vi "TestExplorer.vi"() -> ()   [LabVIEW 2019, in "TestExplorer.lvlib"]
uses:
  TestExplorer.lvlib
  TestResult/TestResult.lvclass
  TestRunner/TestRunner.lvclass
  ResultTreeListener/ResultTreeListener.lvclass
  C:/Users/de200256/Code/neuperger/lvunit/TestListener/TestListener.lvclass
  ResultTree/ResultTree.lvclass
panel:
  out "#Total":i32
  out "#Failed":i32
  out "#Passed":i32
  in  "Result Tree":string(tree)
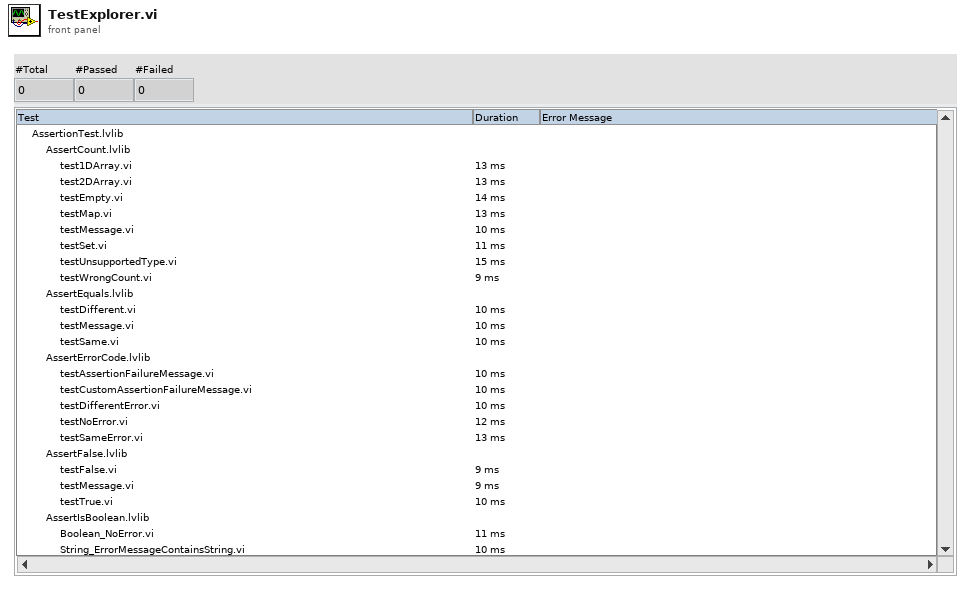
[diagram p1: front panel]
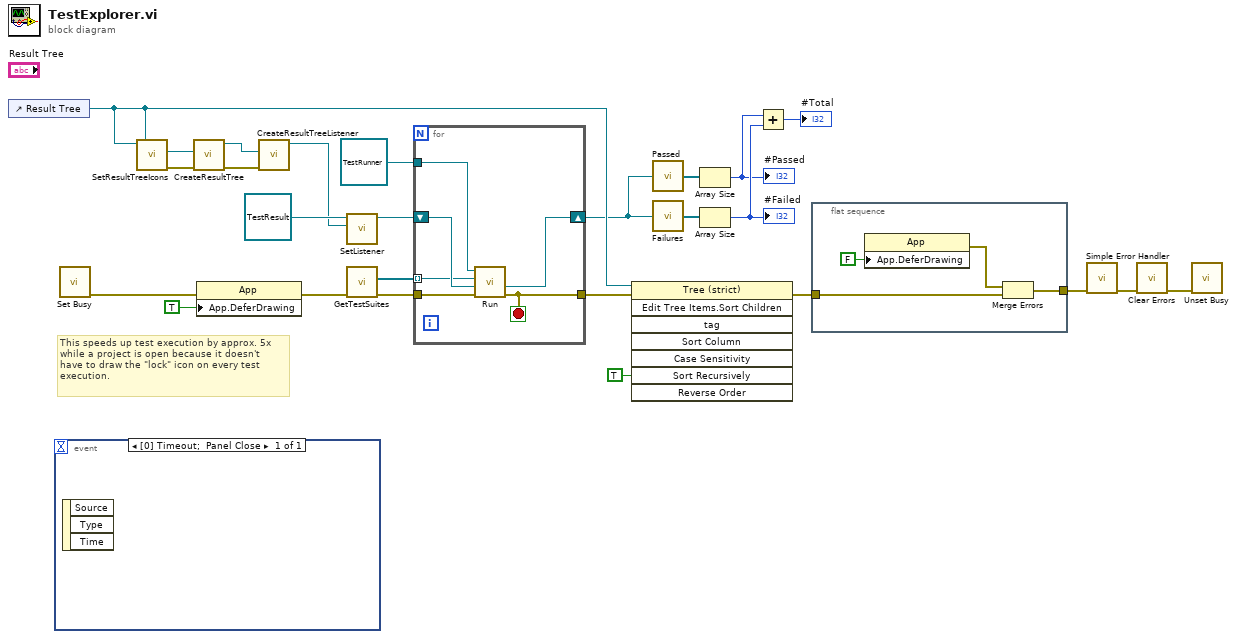
[diagram p0: block diagram]
diagram:
  # "This speeds up test execution by approx. 5x\nwhile a project is open because it doesn't\nhave to draw the \"lock\" icon on every test\nexecution."
  n1 = control-ref of="Result Tree"() -> (w12:refnum<vi>)
  n2 = event shown="[0] Timeout;  Panel Close" {
    selector: _ -> [_]
    dyn-events: _ -> [_]
    timeout: _ -> [_]
    event Timeout; Panel Close {
      n3 = event-data() -> ()  [unwired: 1 in, 3 out]
    }
  }
  n4 = call <vilib>:"Set Busy.vi"() -> ("error out"=w3:errorcluster)  [unwired: 10 in, 1 out]
  n5 = call "SetResultTreeIcons.vi"("Tree Refnum"=w12) -> ("error out"=w14:errorcluster)  [unwired: 10 in]
  n6 = call "CreateResultTree.vi"("error in (no error)"=w14, "Tree Refnum"=w12) -> ("error out"=w19:errorcluster, "ResultTree out"=w21:refnum<class "ResultTree.lvclass">)  [unwired: 8 in]
  n7 = property class="App"(error in=w3, "App.DeferDrawing"=TRUE ("Application:Defer Drawing")) -> (error out=w15:errorcluster)  [unwired: 1 in, 1 out]
  n8 = call "CreateResultTreeListener.vi"("error in (no error)"=w19, "ResultTree"=w21) -> ("ResultTreeListener out"=w20:refnum<class "ResultTreeListener.lvclass">)  [unwired: 8 in, 1 out]
  n9 = call "SetListener.vi"("Listener"=w20, "TestResult in"=refnum<class "TestResult.lvclass"> refnum ("TestResult out")) -> ("TestResult out"=w22:refnum<class "TestResult.lvclass">)  [unwired: 8 in, 1 out]
  n10 = call "GetTestSuites.vi"("error in (no error)"=w15) -> ("error out"=w16:errorcluster, "Tests"=w17:refnum<class "Test.lvclass">[])  [unwired: 9 in]
  n11 = for {
    shift-right: [w30] -> w4
    shift-left: w22 -> [w31]
    tunnel: [w27] -> w13
    tunnel: refnum<class "TestRunner.lvclass"> refnum ("TestRunner in") -> [w29]
    tunnel: w17 -> [w28] mode=indexing
    tunnel: w16 -> [w26]
    stop <- w27 stop-if-true
    n12 = call-dynamic "Run.vi"("error in (no error)"=w26, "TestResult"=w31, "Test"=w28, "TestRunner in"=w29) -> ("error out"=w27:errorcluster, "TestResult out"=w30:refnum<class "TestResult.lvclass">)  [unwired: 5 in, 1 out]
  }
  n13 = invoke class="Tree (strict)" method="Edit Tree Items.Sort Children"(reference=w12, error in=w13, "Sort Recursively"=TRUE ("Sort Recursively?")) -> (error out=w11:errorcluster)  [unwired: 5 in, 7 out]
  n14 = call "Passed.vi"("TestResult In"=w4) -> ("Passed"=w9:refnum<class "Test.lvclass">[])
  n15 = call "Failures.vi"("TestResult In"=w4) -> ("Failures"=w8:refnum<class "TestFailure.lvclass">[])
  n16 = Array Size(array=w9) -> (size(s)=w6:i32)
  "#Passed" <- w6
  n17 = Array Size(array=w8) -> (size(s)=w7:i32)
  "#Failed" <- w7
  n18 = Add(x=w6, y=w7) -> (x+y=→"#Total":i32)
  n19 = flat-sequence {
    tunnel: w11 -> [w34]
    tunnel: [w32] -> w10
    frame #0 {
      n20 = property class="App"("App.DeferDrawing"=FALSE ("Application:Defer Drawing")) -> (error out=w33:errorcluster)  [unwired: 2 in, 1 out]
      n21 = Merge Errors(w33, w34) -> (w32:errorcluster)
    }
  }
  n22 = call <vilib>:"Simple Error Handler.vi"("error in (no error)"=w10) -> ("error out"=w2:errorcluster)  [unwired: 4 in, 4 out]
  n23 = call <vilib>:"Clear Errors.vi"("error in (no error)"=w2) -> ("error out"=w1:errorcluster)  [unwired: 5 in, 1 out]
  n24 = call <vilib>:"Unset Busy.vi"("error in (no error)"=w1) -> ()  [unwired: 10 in, 1 out]
